vi "Pro8000Dump.vi"() -> ()   [LabVIEW 2012]
panel:
  in  "Slot String":string=":SLOT 2"
  in  "Write[T]/Read[F]":bool[](array[boolean])=[FALSE, FALSE, FALSE, FALSE, FALSE, FALSE, FALSE, FALSE, FALSE, FALSE, FALSE, FALSE, FALSE, FALSE, FALSE]
  in  "Array":string[](array[string])=[":TEC?", ":TEMP:SET?", ":SENS?", ":LIMT:SET?", ":SHAREP:SET?", ":SHAREI:SET?", ":SHARED:SET?", ":TWIN:SET?", ":LASER?", ":ILD:SET?", ":LDPOL?", ":LIMC:SET?", ":LIMCP:ACT?", ":MODE?", ":TP?"]
  out "Responses":string[](array[string])=[":TEC ON\n", ":TEMP:SET 2.82507000E+01\n", ":SENS TH\n", ":LIMT:SET 2.00705379E-01\n", ":SHAREP:SET 2.50000000E+00\n", ":SHAREI:SET 2.50000000E+00\n", ":SHARED:SET 2.50000000E+00\n", ":TWIN:SET 1.49987793E+00\n", ":LASER ON\n", ":ILD:SET 9.49999988E-02\n", ":LDPOL CG\n", ":LIMC:SET 1.80088744E-01\n", ":LIMCP:ACT 1.85042575E-01\n", ":MODE CC\n", ":TP ON\n"]
  out "ErrorOut":errorcluster
  in  "ErrorIn":errorcluster
  in  "ResourceString":string="0;GPIB0::10::INSTR"
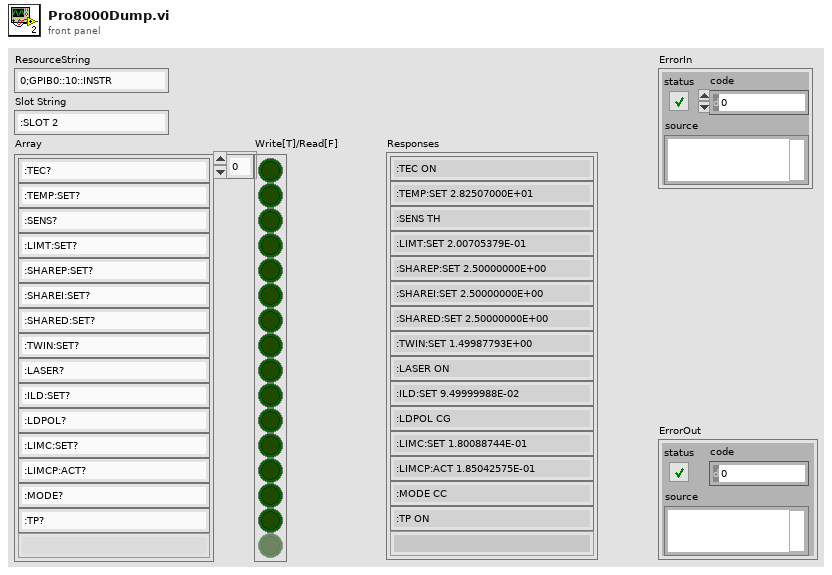
[diagram p1: front panel]
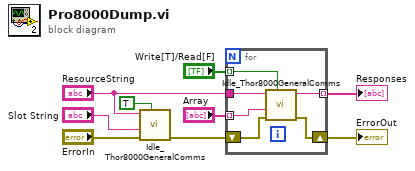
[diagram p0: block diagram]
diagram:
  n1 = call "Idle_Thor8000GeneralComms.vi"("Write[T]/Read[F]"=TRUE, "ErrorIn"="ErrorIn", "Data2Write"="Slot String", "ResourceString"="ResourceString") -> ("ErrorOut"=w4:errorcluster)  [unwired: 6 in, 1 out]
  n2 = for {
    tunnel: "ResourceString" -> [w15]
    shift-right: [w13] -> w9
    shift-left: w4 -> [w14]
    tunnel: [w12] -> w8 mode=indexing
    tunnel: "Write[T]/Read[F]" -> [w11] mode=indexing
    tunnel: "Array" -> [w10] mode=indexing
    n3 = call "Idle_Thor8000GeneralComms.vi"("Write[T]/Read[F]"=w11, "ErrorIn"=w14, "Data2Write"=w10, "ResourceString"=w15) -> ("ErrorOut"=w13:errorcluster, "Response"=w12:string)  [unwired: 6 in]
  }
  "ErrorOut" <- w9
  "Responses" <- w8
